vi "Host.vi"() -> ()   [LabVIEW 2010]
panel:
  in  "stop":bool
  in  "String":string
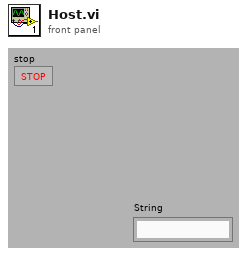
[diagram p1: front panel]
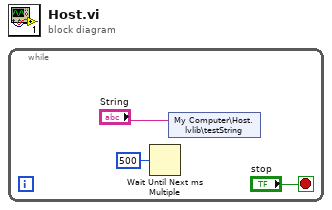
[diagram p0: block diagram]
diagram:
  n1 = while {
    stop <- "stop" stop-if-true
    n2 = Wait Until Next ms Multiple(millisecond multiple=u32 500) -> ()  [unwired: 1 out]
    n3 = shared-variable "My Computer\\Host.lvlib\\testString"("String") -> ()  [unwired: 1 in, 1 out]
  }
